vi "Fdx Set IRIG Time.vi"(8 "error in (no error)":errorcluster, 10 "Irig Time":T1, 11 "InstrumentHandle_board in":u32) -> (0 "error out":errorcluster, 2 "Curent Irig Time":T1, 3 "InstrumentHandle_board out":u32)   [LabVIEW 2020, in "AIM664LV.lvlib"]
uses:
  AIM664LV.lvlib
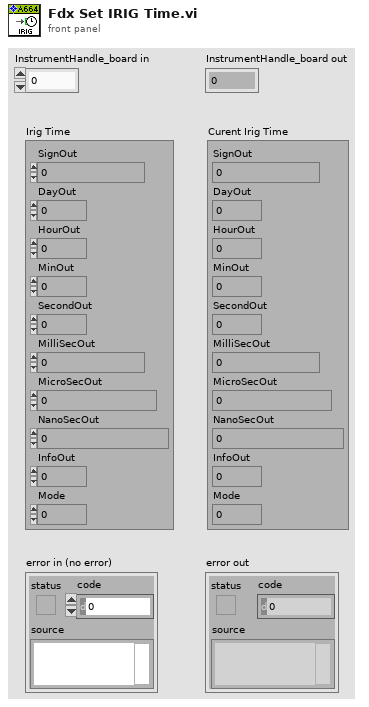
[diagram p1: front panel]
types:
  T1 = cluster{"SignOut":i32, "DayOut":u32, "HourOut":u32, "MinOut":u32, "SecondOut":u32, "MilliSecOut":u32, "MicroSecOut":u32, "NanoSecOut":u32, "InfoOut":u32, "Mode":u32}
  T2 = cluster{"Control":u32, "SignIn":i32, "DayIn":u32, "HourIn":u32, "MinIn":u32, "SecondIn":u32, "MilliSecIn":u32, "MicroSecIn":u32, "NanoSecIn":u32, "InfoIn":u32}
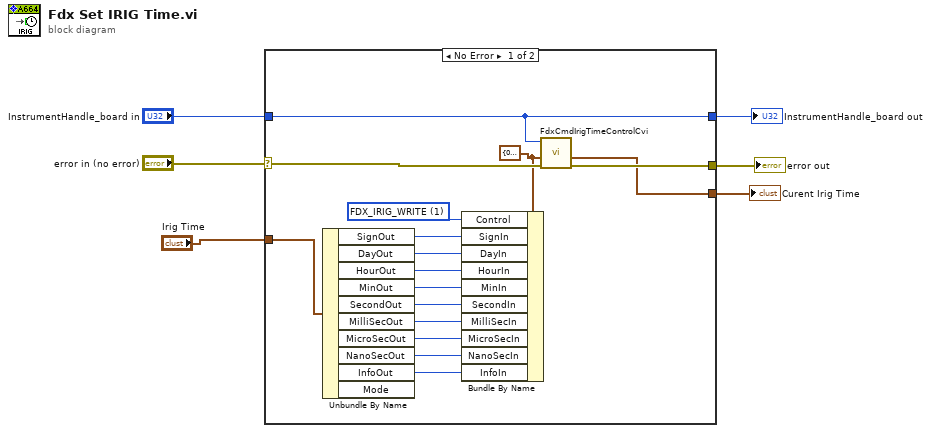
[diagram p0: block diagram]
diagram:
  n1 = case shown="No Error" "error in (no error)" {
    selector: "error in (no error)" -> [w22 w24]
    tunnel: [w21 w24] -> w5
    tunnel: [w19 w23] -> w3
    tunnel: "InstrumentHandle_board in" -> [w19 w23]
    tunnel: [w20 _] -> w2
    tunnel: "Irig Time" -> [w16 _]
    frame No Error {
      w17 = u32 1 items=["FDX_IRIG_READ", "FDX_IRIG_WRITE", "FDX_IRIG_EXTERN", "FDX_IRIG_INTERN"] ("Control")
      w18 = T2 {"Control"=0, "SignIn"=0, "DayIn"=0, "HourIn"=0, "MinIn"=0, "SecondIn"=0, "MilliSecIn"=0, "MicroSecIn"=0, "NanoSecIn"=0, "InfoIn"=0} ("Irig In")
      n2 = Unbundle By Name(w16) -> ("SignOut"=w15:i32, "DayOut"=w14:u32, "HourOut"=w13:u32, "MinOut"=w12:u32, "SecondOut"=w11:u32, "MilliSecOut"=w10:u32, "MicroSecOut"=w9:u32, "NanoSecOut"=w8:u32, "InfoOut"=w7:u32)  [unwired: 1 out]
      n3 = Bundle By Name(cluster=w18, "Control"=w17, "SignIn"=w15, "DayIn"=w14, "HourIn"=w13, "MinIn"=w12, "SecondIn"=w11, "MilliSecIn"=w10, "MicroSecIn"=w9, "NanoSecIn"=w8, "InfoIn"=w7) -> ()  [unwired: 1 out]
      n4 = call "FdxCmdIrigTimeControlCvi.vi"("error in"=w22, "Irig In"=w18, "InstrumentHandle_board in"=w19) -> ("error out"=w21:errorcluster, "Irig Out"=w20:T1)  [unwired: 6 in, 1 out]
    }
    frame Error {
    }
  }
  "error out" <- w5
  "InstrumentHandle_board out" <- w3
  "Curent Irig Time" <- w2
